vi "index.vi"   [LabVIEW 2020]
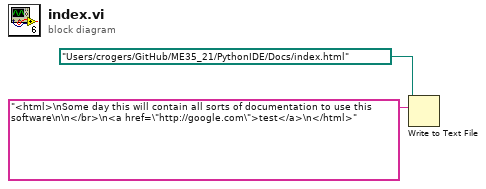
[diagram p0: block diagram]
diagram:
  n1 = Write to Text File(file (use dialog)=path "/Users/crogers/GitHub/ME35_21/PythonIDE/Docs/index.html", text="<html>\nSome day this will contain all sorts of documentation to use this software\n\n</br>\n<a href=\"http://google.com\">test</a>\n</html>") -> ()  [unwired: 2 in, 3 out]
